vi "sub_SDR_mimo_AddSynch.vi"(10 "In frame":cdb[][](array[numeric]), 11 "Synch. Sequence":cdb[](array[numeric])) -> (2 "Output frame":cdb[][](array[numeric]))   [LabVIEW 2012]
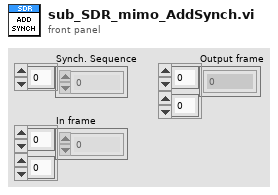
[diagram p1: front panel]
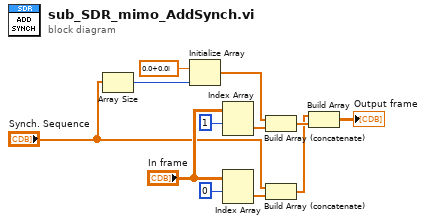
[diagram p0: block diagram]
diagram:
  n1 = Array Size(array="Synch. Sequence") -> (size(s)=w2:i32)
  n2 = Initialize Array(cdb 0.0+0.0i ("element"), w2) -> (w10:cdb[])
  n3 = Index Array(array="In frame", index (row)=1) -> (element=w9:cdb[])  [unwired: 1 in]
  n4 = Index Array(array="In frame", index (row)=0) -> (element=w5:cdb[])  [unwired: 1 in]
  n5 = Build Array (concatenate)(w10, w9) -> (w11:cdb[])
  n6 = Build Array (concatenate)("Synch. Sequence", w5) -> (w1:cdb[])
  n7 = Build Array(w1, w11) -> (→"Output frame":cdb[][])
